vi "Read_Write_Template.vi"(0 "Template File":path, 1 "Mode":T1, 5 "Channel names In":string[](array[string]), 7 "Single Value In":string, 9 "2D Info In":string[][](array[string]), 11 "1D Info In":string[](array[string]), 12 "Save file":bool=TRUE, 13 "Data type":string="Tolerance") -> (3 "Freshly Loaded?":bool, 4 "Template File Out":path, 6 "Template Ch Names Out":string[](array[string]), 8 "Single Value Out":string, 10 "2D Info Out":string[][](array[string]), 14 "Template Info":string[][](array[string]), 15 "1D Info Out":string[](array[string]))   [LabVIEW 2011]
uses:
  Controls/Global_mode.ctl
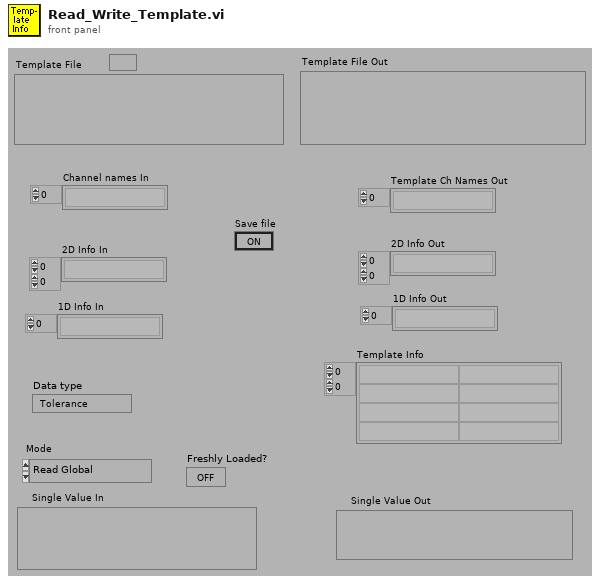
[diagram p1: front panel]
types:
  T1 = typedef "Global_mode.ctl" = enum16{"Read Global", "Load Global From File", "Write Global to File"}
  T2 = typedef "File_Status.ctl" = enum16{"Invalid Path", "This is a folder pathname", "Generic File Error", "Directory structure cannot be created", "File cannot be created", "File can be created", "File exist but read only", "File exist but no access", "File exist with read and write access"}
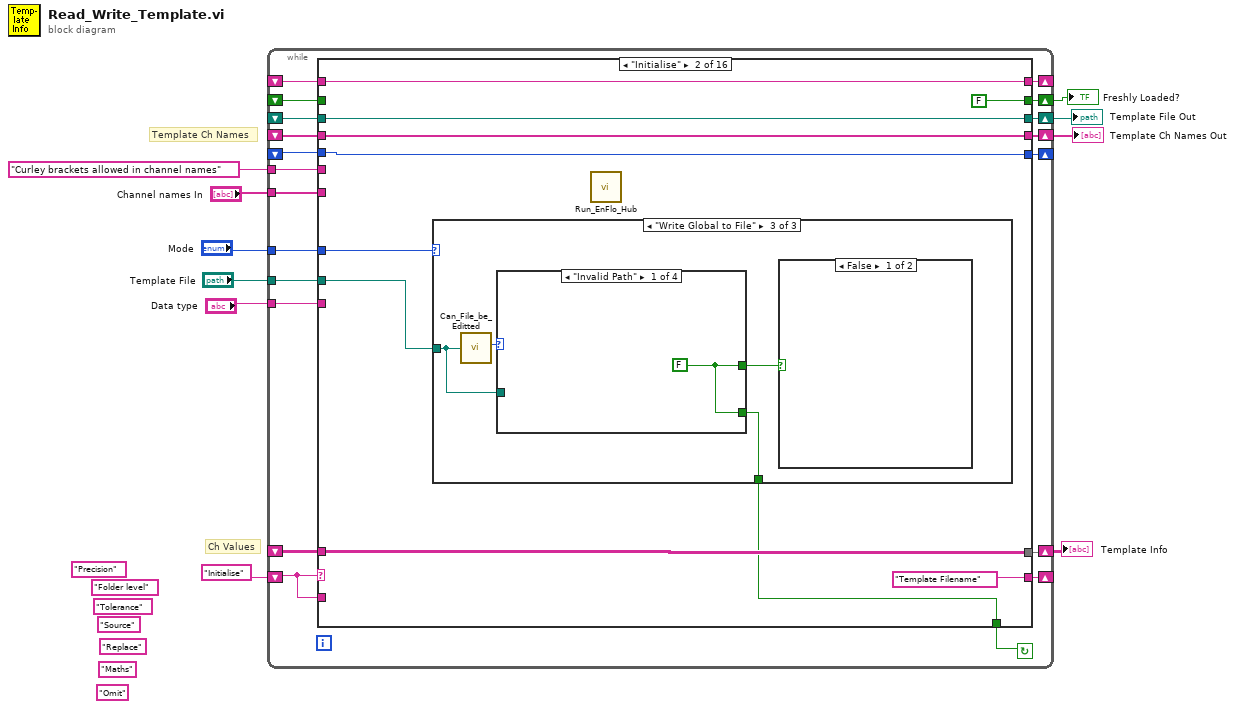
[diagram p0: block diagram]
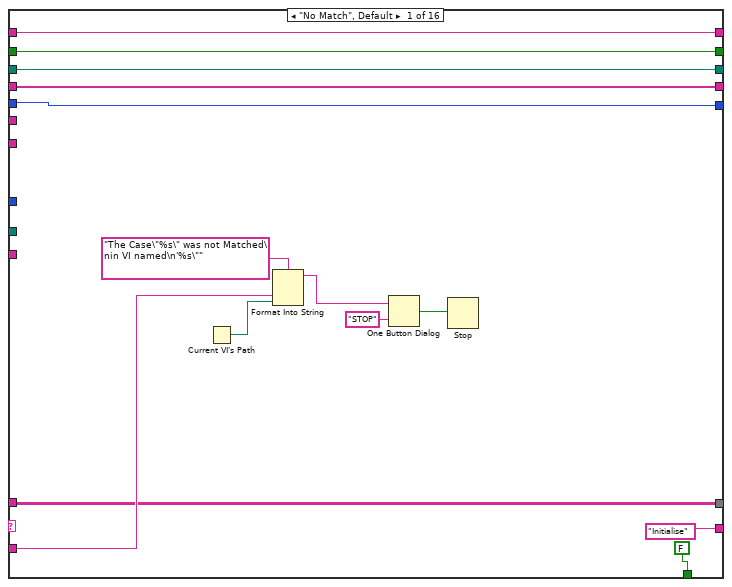
[diagram p2: hidden frame]
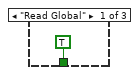
[diagram p3: hidden frame]
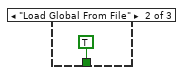
[diagram p4: hidden frame]
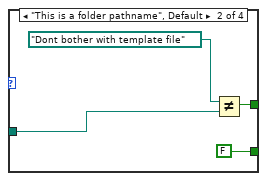
[diagram p5: hidden frame]
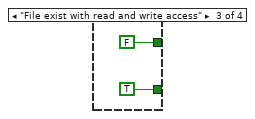
[diagram p6: hidden frame]
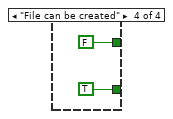
[diagram p7: hidden frame]
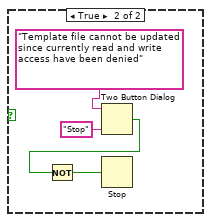
[diagram p8: hidden frame]
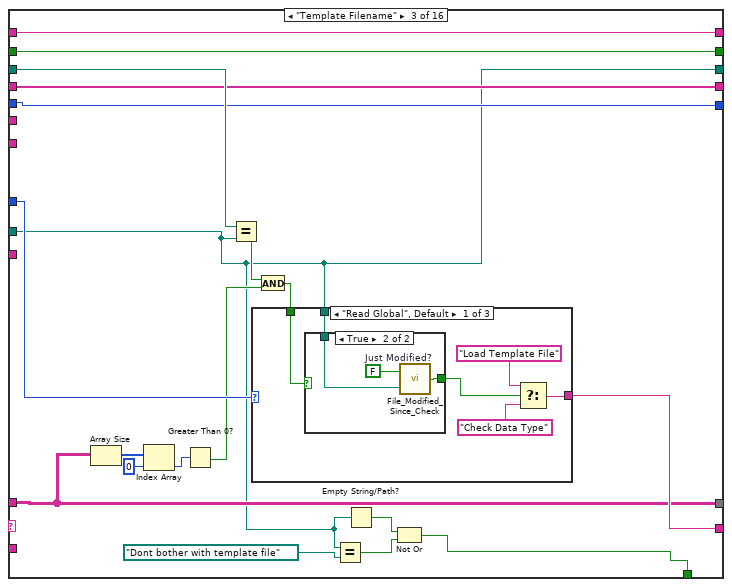
[diagram p9: hidden frame]
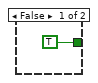
[diagram p10: hidden frame]
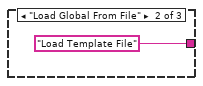
[diagram p11: hidden frame]
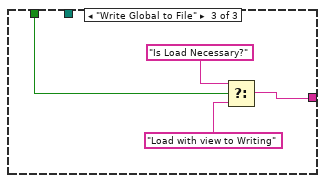
[diagram p12: hidden frame]
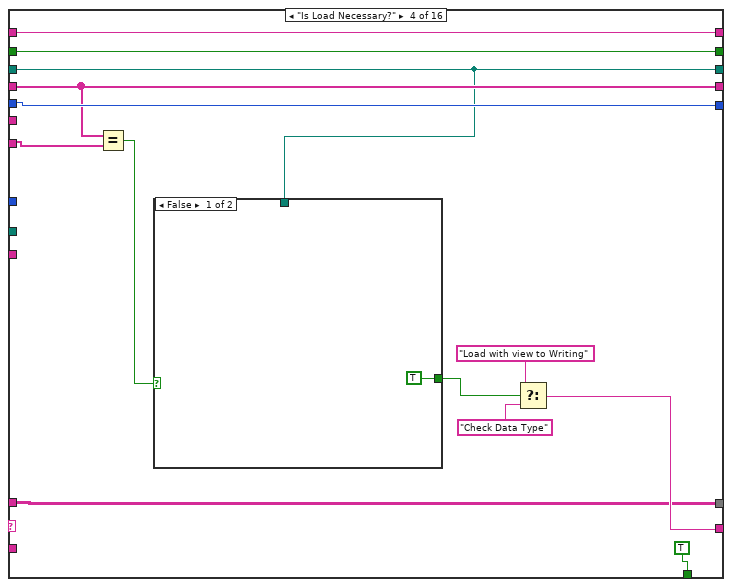
[diagram p13: hidden frame]
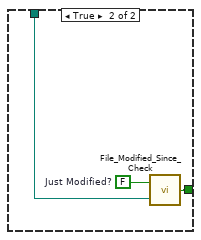
[diagram p14: hidden frame]
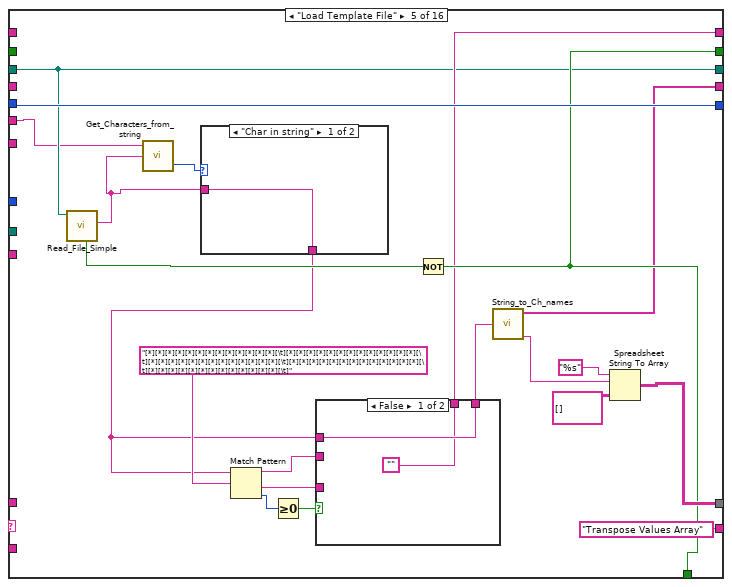
[diagram p15: hidden frame]
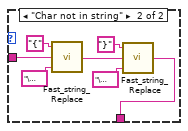
[diagram p16: hidden frame]
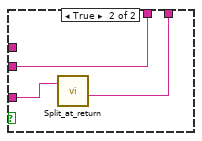
[diagram p17: hidden frame]
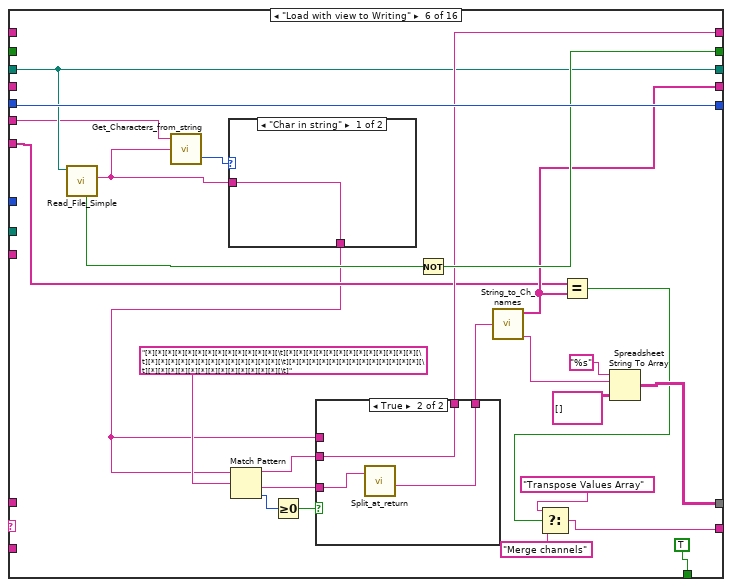
[diagram p18: hidden frame]
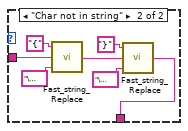
[diagram p19: hidden frame]
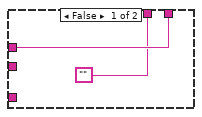
[diagram p20: hidden frame]
diagram:
  (unwired) "Precision"
  (unwired) "Folder level"
  (unwired) "Omit"
  (unwired) "Maths"
  (unwired) "Tolerance"
  (unwired) "Source"
  (unwired) "Replace"
  # "Template Ch Names"
  # "Ch Values"
  n1 = while {
    shift-left: _ -> [w15]
    shift-right: [w16] -> w3
    tunnel: "Channel names In" -> [w18]
    shift-left: _ -> [w17]
    shift-right: [w19] -> _
    tunnel: "Data type" -> [w20]
    shift-left: _ -> [w21]
    shift-right: [w22] -> w6
    shift-left: _ -> [w25]
    shift-right: [w24] -> w7
    shift-left: _ -> [w26]
    shift-right: [w27] -> w8
    tunnel: "Mode" -> [w28]
    shift-left: "Initialise" -> [w23]
    shift-right: [w29] -> _
    shift-right: [w14] -> _
    shift-left: _ -> [w13]
    tunnel: "Template File" -> [w12]
    tunnel: "Curley brackets allowed in channel names" -> [w11]
    stop <- w30 continue-if-true
    n2 = case shown="\"Initialise\"" w23 {
      tunnel: [FALSE w45 w75 TRUE w138 TRUE ("Save file") TRUE ("Save file") TRUE w243 FALSE FALSE FALSE "Save file" FALSE ("Save file") w472 FALSE] -> w30
      tunnel: ["Initialise" "Template Filename" w89 w120 "Transpose Values Array" w166 "Transpose Values Array" "Check Data Type" w240 "" "" "" "Save Template File" "End" w469 "End"] -> w29
      tunnel: w28 -> [_ w47 w90 _ _ _ _ _ w242 _ _ _ _ _ _ _]
      tunnel: [w35 w53 w85 w114 w142 w182 w203 w230 w246 w310 w324 w344 w370 w457 w467 w526] -> w27
      tunnel: w26 -> [w35 w53 w85 w114 _ _ w201 w229 w246 w310 w324 w344 w371 w457 w466 w526]
      tunnel: w25 -> [w37 w54 w92 w110 w130 w163 w206 w225 w245 w312 w330 w346 w372 w451 w471 w525]
      tunnel: [w37 w54 w74 w110 w130 w163 w206 w225 w245 w312 w330 w346 w372 w451 w471 w525] -> w24
      tunnel: w23 -> [w39 _ _ _ _ _ _ _ _ _ _ _ _ _ _ _]
      tunnel: [w38 w52 w91 w113 w129 w170 w205 w224 w244 w308 w325 w341 w365 w460 w470 w524] -> w22
      tunnel: w21 -> [w38 w52 w91 w113 _ _ w204 w224 w244 w308 w325 w341 w365 w460 w470 w524]
      tunnel: w20 -> [_ _ _ _ _ _ _ _ w247 w311 w322 w345 w368 w453 _ _]
      tunnel: [w33 w50 w84 w118 w144 w184 w209 w223 w241 w301 w327 w333 w363 w459 w468 w522] -> w19
      tunnel: w18 -> [_ _ _ w112 _ w169 w205 _ _ w302 _ w338 w364 _ _ _]
      tunnel: w17 -> [w33 w50 w84 w118 w144 w184 w209 w223 _ w301 w327 w333 w363 w459 w468 w522]
      tunnel: [w32 FALSE w80 w109 w138 w178 w207 w221 w239 w300 w326 w332 w362 w458 w465 w520] -> w16
      tunnel: w15 -> [w32 _ w80 w109 _ _ w207 w221 w239 w300 w326 w332 w362 w458 w465 w520]
      tunnel: [w31 w48 w79 w108 w132 w172 w208 w220 w238 w299 w323 w331 w360 w455 w463 w519] -> w14
      tunnel: w13 -> [w31 w48 w79 w108 _ _ w208 w220 w238 w299 w323 w331 w360 w454 w464 w519]
      tunnel: w12 -> [_ w46 w74 _ _ _ _ _ _ _ _ _ _ _ _ _]
      tunnel: w11 -> [_ _ _ _ w126 w162 _ _ _ _ _ _ _ _ w462 _]
      frame "No Match", Default {
        n3 = Current VI's Path() -> (path=w40:path)
        n4 = Format Into String(format string="The Case\"%s\" was not Matched\nin VI named\n'%s\"" ("Format String"), w39, w40) -> (resulting string=w43:string)  [unwired: 2 in, 1 out]
        n5 = One Button Dialog(message=w43, button name ("OK")="STOP") -> (true=w41:bool)
        n6 = Stop(stop? (T)=w41) -> ()
      }
      frame "Initialise" {
        n7 = case shown="\"Write Global to File\"" w47 {
          tunnel: w46 -> [_ _ w57]
          tunnel: [TRUE TRUE w58] -> w45
          frame "Read Global" {
          }
          frame "Load Global From File" {
          }
          frame "Write Global to File" {
            n8 = call "Can_File_be_Editted.vi"("Filename"=w57) -> ("File Status"=w60:T2)  [unwired: 3 out]
            n9 = case shown="\"Invalid Path\"" w60 {
              tunnel: [w61 w63 FALSE FALSE] -> w59
              tunnel: [w61 FALSE TRUE TRUE] -> w58
              tunnel: w57 -> [_ w62 _ _]
              frame "Invalid Path" {
                w61 = FALSE
              }
              frame "This is a folder pathname", Default {
                n10 = Not Equal?(x=path "Dont bother with template file" ("Template File"), y=w62) -> (x != y?=w63:bool)
              }
              frame "File exist with read and write access" {
              }
              frame "File can be created" {
              }
            }
            n11 = case shown="False" w59 {
              frame False {
              }
              frame True {
                n12 = Two Button Dialog(message="Template file cannot be updated since currently read and write access have been denied", 1:"Stop" ("F button name (\"Cancel\")")) -> (T button?=w71:bool)  [unwired: 1 out]
                n13 = Not(x=w71) -> (.not. x?=w70:bool)
                n14 = Stop(stop? (T)=w70) -> ()
              }
            }
          }
        }
        n15 = call "Run_EnFlo_Hub.vi"() -> ()  [unwired: 8 out]
      }
      frame "Template Filename" {
        n16 = Array Size(array=w85) -> (size(s)=w86:i32[])
        n17 = Index Array(array=w86, index=0 ("Index")) -> (element=w88:i32)
        n18 = Greater Than 0?(x=w88) -> (x > 0?=w81:bool)
        n19 = Equal?(x=w92, y=w74) -> (x = y?=w83:bool)
        n20 = And(x=w83, y=w81) -> (x .and. y?=w82:bool)
        n21 = case shown="\"Read Global\", Default" w90 {
          tunnel: w82 -> [w98 _ w107]
          tunnel: [w94 "Load Template File" w105] -> w89
          tunnel: w74 -> [w97 _ _]
          frame "Read Global", Default {
            n22 = case shown="True" w98 {
              tunnel: w97 -> [_ w102]
              tunnel: [TRUE ("Modified?") w101] -> w96
              frame False {
              }
              frame True {
                w100 = FALSE  # Just Modified?
                n23 = call "File_Modified_Since_Check.vi"("Pathname"=w102, "Just Modified?"=w100) -> ("Modified?"=w101:bool)
              }
            }
            n24 = Select(t="Load Template File", s=w96, f="Check Data Type") -> (s? t:f=w94:string)
          }
          frame "Load Global From File" {
          }
          frame "Write Global to File" {
            n25 = Select(t="Is Load Necessary?", s=w107, f="Load with view to Writing") -> (s? t:f=w105:string)
          }
        }
        n26 = Equal?(x=w74, y=path "Dont bother with template file" ("Template File")) -> (x = y?=w77:bool)
        n27 = Empty String/Path?(string/path=w74) -> (empty?=w76:bool)
        n28 = Not Or(1:w77, 2:w76) -> (0:w75:bool)
      }
      frame "Is Load Necessary?" {
        n29 = Equal?(x=w113, y=w112) -> (x = y?=w111:bool)
        n30 = case shown="False" w111 {
          tunnel: w110 -> [_ w124]
          tunnel: [TRUE ("Modified?") w123] -> w117
          frame False {
          }
          frame True {
            w122 = FALSE  # Just Modified?
            n31 = call "File_Modified_Since_Check.vi"("Pathname"=w124, "Just Modified?"=w122) -> ("Modified?"=w123:bool)
          }
        }
        n32 = Select(t="Load with view to Writing", s=w117, f="Check Data Type") -> (s? t:f=w120:string)
      }
      frame "Load Template File" {
        n33 = call "Read_File_Simple.vi"("Filename"=w130) -> ("Error?"=w143:bool, "string"=w127:string)  [unwired: 2 in, 6 out]
        n34 = call "Get_Characters_from_string.vi"("Input string"=w127, "Variable name"=w126) -> ("Status"=w128:enum16{"Char in string", "Char not in string"})  [unwired: 1 in, 1 out]
        n35 = case shown="\"Char in string\"" w128 {
          tunnel: w127 -> [w146 w152]
          tunnel: [w146 w147] -> w125
          frame "Char in string" {
          }
          frame "Char not in string" {
            n36 = call "Fast_string_Replace.vi"("Replace match with:"="\u0002" ("regular expression"), "Input String"=w152, "regular expression"="{") -> ("Output String"=w148:string)  [unwired: 2 out]
            n37 = call "Fast_string_Replace.vi"("Replace match with:"="\u0003" ("regular expression"), "Input String"=w148, "regular expression"="}") -> ("Output String"=w147:string)  [unwired: 2 out]
          }
        }
        n38 = Match Pattern(string=w125, regular expression="[*][*][*][*][*][*][*][*][*][*][*][*][*][\t][*][*][*][*][*][*][*][*][*][*][*][*][*][\t][*][*][*][*][*][*][*][*][*][*][*][*][*][\t][*][*][*][*][*][*][*][*][*][*][*][*][*][\t][*][*][*][*][*][*][*][*][*][*][*][*][*][\t]" ("String")) -> (before substring=w131:string, after substring=w136:string, offset past match=w135:i32)  [unwired: 2 out]
        n39 = Greater Or Equal To 0?(x=w135) -> (x >= 0?=w134:bool)
        n40 = case shown="False" w134 {
          tunnel: w136 -> [_ w158]
          tunnel: [w155 w157] -> w133
          tunnel: w125 -> [w155 _]
          tunnel: ["" w156] -> w132
          tunnel: w131 -> [_ w156]
          frame False {
          }
          frame True {
            n41 = call "Split_at_return.vi"("String"=w158) -> ("after substring"=w157:string)  [unwired: 1 in, 3 out]
          }
        }
        n42 = Not(x=w143) -> (.not. x?=w138:bool)
        n43 = call "String_to_Ch_names.vi"("Spreadsheet string"=w133) -> ("Ch names"=w129:string[], "String After names"=w139:string)  [unwired: 2 out]
        n44 = Spreadsheet String To Array(format string="%s", spreadsheet string=w139, array type (2D Dbl)=string[][] [] ("Channel Values")) -> (array=w142:string[][])  [unwired: 1 out]
      }
      frame "Load with view to Writing" {
        n45 = call "Read_File_Simple.vi"("Filename"=w163) -> ("Error?"=w183:bool, "string"=w160:string)  [unwired: 2 in, 6 out]
        n46 = call "Get_Characters_from_string.vi"("Input string"=w160, "Variable name"=w162) -> ("Status"=w161:enum16{"Char in string", "Char not in string"})  [unwired: 1 in, 1 out]
        n47 = case shown="\"Char in string\"" w161 {
          tunnel: w160 -> [w185 w191]
          tunnel: [w185 w186] -> w159
          frame "Char in string" {
          }
          frame "Char not in string" {
            n48 = call "Fast_string_Replace.vi"("Replace match with:"="\u0002" ("regular expression"), "Input String"=w191, "regular expression"="{") -> ("Output String"=w187:string)  [unwired: 2 out]
            n49 = call "Fast_string_Replace.vi"("Replace match with:"="\u0003" ("regular expression"), "Input String"=w187, "regular expression"="}") -> ("Output String"=w186:string)  [unwired: 2 out]
          }
        }
        n50 = Match Pattern(string=w159, regular expression="[*][*][*][*][*][*][*][*][*][*][*][*][*][\t][*][*][*][*][*][*][*][*][*][*][*][*][*][\t][*][*][*][*][*][*][*][*][*][*][*][*][*][\t][*][*][*][*][*][*][*][*][*][*][*][*][*][\t][*][*][*][*][*][*][*][*][*][*][*][*][*][\t]" ("String")) -> (before substring=w171:string, after substring=w176:string, offset past match=w175:i32)  [unwired: 2 out]
        n51 = Greater Or Equal To 0?(x=w175) -> (x >= 0?=w174:bool)
        n52 = case shown="True" w174 {
          tunnel: w176 -> [_ w197]
          tunnel: [w194 w196] -> w173
          tunnel: w159 -> [w194 _]
          tunnel: ["" w195] -> w172
          tunnel: w171 -> [_ w195]
          frame False {
          }
          frame True {
            n53 = call "Split_at_return.vi"("String"=w197) -> ("after substring"=w196:string)  [unwired: 1 in, 3 out]
          }
        }
        n54 = Not(x=w183) -> (.not. x?=w178:bool)
        n55 = call "String_to_Ch_names.vi"("Spreadsheet string"=w173) -> ("Ch names"=w170:string[], "String After names"=w179:string)  [unwired: 2 out]
        n56 = Equal?(x=w169, y=w170) -> (x = y?=w168:bool)
        n57 = Select(t="Transpose Values Array", s=w168, f="Merge channels") -> (s? t:f=w166:string)
        n58 = Spreadsheet String To Array(format string="%s", spreadsheet string=w179, array type (2D Dbl)=string[][] [] ("Channel Values")) -> (array=w182:string[][])  [unwired: 1 out]
      }
      frame "Merge channels" {
        n59 = Array Size(array=w201) -> (size(s)=w200:i32[])
        n60 = Index Array(array=w200, index=0) -> (element=w198:i32)
        n61 = case shown="1, Default" w198 {
          tunnel: w205 -> [w212 w219]
          tunnel: w204 -> [_ w218]
          tunnel: w201 -> [_ w217]
          tunnel: [w211 w216] -> w203
          frame 0 {
            n62 = Array Size(array=w212) -> (size(s)=w213:i32)
            n63 = Initialize Array("", 0 ("Dimension Size"), w213) -> (w211:string[][])
          }
          frame 1, Default {
            n64 = call "Merge_2D_values.vi"("Values In"=w217, "Present Channels"=w218, "Desired Channels"=w219) -> ("Values Out"=w216:string[][])
          }
        }
      }
      frame "Transpose Values Array" {
        n65 = Array Size(array=w229) -> (size(s)=w227:i32[])
        n66 = Index Array(array=w227, index=1 ("Index")) -> (element=w226:i32)
        n67 = for {
          N: w226 -> [_]
          tunnel: w229 -> [w234]
          tunnel: [w235] -> w230 mode=indexing
          i -> [w233]
          n68 = Index Array(array=w234, index (col)=w233) -> (element=w232:string[])  [unwired: 1 in]
          n69 = for {
            tunnel: [w237] -> w235 mode=indexing
            tunnel: w232 -> [w236] mode=indexing
            n70 = call "Remove_Quotes.vi"("String"=w236) -> ("String Out"=w237:string)
          }
        }
      }
      frame "Check Data Type" {
        n71 = case shown="\"Precision\"" w247 {
          tunnel: [1 1 1 1 1 2 1 1 2 2 2 1 2 1 1 0] -> w241
          tunnel: w247 -> [w258 _ _ _ _ _ _ _ _ _ _ _ _ _ _ _]
          tunnel: [w257 TRUE TRUE TRUE TRUE TRUE TRUE TRUE TRUE TRUE TRUE TRUE TRUE TRUE TRUE TRUE] -> w243
          frame "No Match", Default {
            n72 = Empty String/Path?(string/path=w258) -> (empty?=w259:bool)
            n73 = case shown="False" w259 {
              tunnel: w258 -> [w262 _]
              tunnel: [FALSE FALSE] -> w257
              frame False {
                n74 = Current VI's Path() -> (path=w263:path)
                n75 = Format Into String(format string="The Case\"%s\" was not Matched\nin VI named\n'%s\"" ("Format String"), w262, w263) -> (resulting string=w266:string)  [unwired: 2 in, 1 out]
                n76 = One Button Dialog(message=w266, button name ("OK")="STOP") -> (true=w264:bool)
                n77 = Stop(stop? (T)=w264) -> ()
              }
              frame True {
              }
            }
          }
          frame "Description" {
          }
          frame "Dispose" {
          }
          frame "Decimal" {
          }
          frame "Precision" {
          }
          frame "Multiple Sources" {
          }
          frame "Summarise" {
          }
          frame "Tolerance" {
          }
          frame "Source" {
          }
          frame "Replace" {
          }
          frame "Ignore When" {
          }
          frame "Maths" {
          }
          frame "Omit" {
          }
          frame "Folder level" {
          }
          frame "Minimum Value" {
          }
          frame "Log Folder Name" {
          }
        }
        n78 = case shown="\"Write Global to File\"" w242 {
          tunnel: w241 -> [w249 w253]
          tunnel: [w248 w254] -> w240
          frame "Read Global", Default {
            n79 = case shown="0" w249 {
              tunnel: ["Create Outputs 2D" "Create Outputs 1D" "Create single value output"] -> w248
              frame 2, Default {
              }
              frame 1 {
              }
              frame 0 {
              }
            }
          }
          frame "Write Global to File" {
            n80 = case shown="0" w253 {
              tunnel: ["Replace single value" "Replace Values"] -> w254
              frame 0 {
              }
              frame 1, Default {
              }
            }
          }
        }
      }
      frame "Create Outputs 1D" {
        n81 = for {
          tunnel: w311 -> [w320]
          tunnel: w310 -> [w319] mode=indexing
          tunnel: [w318] -> w309 mode=indexing
          n82 = call "Get_Array_Subset.vi"("String Array In"=w319, "Subset Name"=w320) -> ("First Element"=w318:string)  [unwired: 4 out]
        }
        n83 = Array Size(array=w302) -> (size(s)=w304:i32)
        n84 = Equal To 0?(x=w304) -> (x = 0?=w303:bool)
        n85 = case shown="False" w303 {
          tunnel: w309 -> [w316 w317]
          tunnel: w302 -> [w315 _]
          tunnel: w308 -> [w314 _]
          tunnel: [w313 w317] -> w307
          frame False {
            n86 = call "Merge_row_values.vi"("Present Row values"=w316, "Present Channels"=w314, "Desired Channels"=w315) -> ("Desired Row values"=w313:string[])  [unwired: 1 out]
          }
          frame True {
          }
        }
        "1D Info Out" <- w307
      }
      frame "Create single value output" {
        n87 = call "Get_Characters_from_string.vi"("Input string"=w323, "Variable name"=w322) -> ("Value"=→"Single Value Out":string)  [unwired: 1 in, 1 out]
      }
      frame "Create Outputs 2D" {
        n88 = for {
          tunnel: w345 -> [w359]
          tunnel: w344 -> [w358] mode=indexing
          tunnel: [w357] -> w340 mode=indexing
          n89 = call "Get_Array_Subset.vi"("String Array In"=w358, "Subset Name"=w359) -> ("Array Subset Out"=w357:string[])  [unwired: 4 out]
        }
        n90 = Equal?(x=w341, y=w338) -> (x = y?=w336:bool)
        n91 = Array Size(array=w338) -> (size(s)=w337:i32)
        n92 = Equal To 0?(x=w337) -> (x = 0?=w335:bool)
        n93 = Or(x=w336, y=w335) -> (x .or. y?=w334:bool)
        n94 = case shown="False" w334 {
          tunnel: w341 -> [w350 _]
          tunnel: w338 -> [w349 _]
          tunnel: w340 -> [w348 w356]
          tunnel: [w347 w356] -> w339
          frame False {
            n95 = for {
              tunnel: w350 -> [w355]
              tunnel: w349 -> [w354] mode=indexing
              tunnel: w348 -> [w352]
              tunnel: [w351] -> w347 mode=indexing
              n96 = Search 1D Array(1D array=w355, element=w354) -> (index of element=w353:i32)  [unwired: 1 out]
              n97 = Index Array(array=w352, index (row)=w353) -> (element=w351:string[])  [unwired: 1 in]
            }
          }
          frame True {
          }
        }
        "2D Info Out" <- w339
      }
      frame "Replace Values" {
        n98 = for {
          tunnel: w368 -> [w381]
          tunnel: w371 -> [w380] mode=indexing
          tunnel: [w379] -> w370 mode=indexing
          tunnel: w365 -> [w378] mode=indexing
          tunnel: w363 -> [w377]
          tunnel: "1D Info In" -> [w376]
          tunnel: "2D Info In" -> [w375]
          tunnel: w365 -> [w374] mode=indexing
          tunnel: w364 -> [w373]
          n99 = stacked-sequence {
            seq-local: [_ w391 _ _ _] -> [_ _ _ w442 _]
            seq-local: [_ w390 _ _ _] -> [_ _ _ w443 _]
            seq-local: [_ _ w402 _ _] -> [_ _ _ w441 _]
            seq-local: [_ w389 _ _ _] -> [_ _ w398 _ _]
            seq-local: [w384 _ _ _ _] -> [_ _ w399 _ _]
            seq-local: [w382 _ _ _ _] -> [_ _ w397 _ _]
            tunnel: w381 -> [_ w396 _ w444 _]
            tunnel: w380 -> [_ w393 _ _ _]
            tunnel: [_ _ _ w434 _] -> w379
            tunnel: w378 -> [_ _ _ w435 _]
            tunnel: w377 -> [w383 _ _ _ _]
            tunnel: w376 -> [_ _ w401 _ _]
            tunnel: w375 -> [_ _ w400 _ _]
            tunnel: w374 -> [w386 _ _ _ _]
            tunnel: w373 -> [w385 _ _ _ _]
            frame #0 {
              n100 = Search 1D Array(1D array=w385, element=w386) -> (index of element=w382:i32)  [unwired: 1 out]
              n101 = case shown="-1" w382 {
                tunnel: [w387 0] -> w384
                tunnel: w383 -> [w387 _]
                frame 0, Default {
                }
                frame -1 {
                }
              }
            }
            frame #1 {
              n102 = call "Get_Array_Subset.vi"("String Array In"=w393, "Subset Name"=w396) -> ("index after match"=w392:i32, "Array Subset Out"=w389:string[], "Length before match"=w394:i32)  [unwired: 2 out]
              n103 = Array Subset(array=w393, index=0 ("Array Index"), length=w394) -> (w391:string[])
              n104 = Array Subset(array=w393, index=w392) -> (w390:string[])  [unwired: 1 in]
            }
            frame #2 {
              n105 = case shown="2, Default" w399 {
                tunnel: [w406 w430 w433] -> w402
                tunnel: w401 -> [_ w432 _]
                tunnel: w400 -> [w405 _ _]
                tunnel: w398 -> [_ _ w433]
                tunnel: w397 -> [w403 w429 _]
                frame 2, Default {
                  n106 = Index Array(array=w405, index (row)=w403) -> (element=w404:string[])  [unwired: 1 in]
                  n107 = while {
                    shift-left: _ -> [w407]
                    shift-right: [w408] -> _
                    tunnel: [w409] -> w406
                    tunnel: w404 -> [w411]
                    i -> [w412]
                    stop <- w410 continue-if-true
                    n108 = case shown="0, Default" w412 {
                      tunnel: w411 -> [w414 w417]
                      tunnel: [w415 FALSE] -> w410
                      tunnel: [w414 w420] -> w409
                      tunnel: [w413 w419] -> w408
                      tunnel: w407 -> [_ w419]
                      frame 0, Default {
                        n109 = Empty String/Path?(string/path=w414) -> (empty?=w413:bool[])
                        n110 = Or Array Elements(Boolean array=w413) -> (logical OR=w415:bool)
                      }
                      frame 1 {
                        n111 = for {
                          shift-right: [w423] -> w420
                          shift-left: string[] [] -> [w422]
                          tunnel: w419 -> [w424] mode=indexing
                          tunnel: w417 -> [w421] mode=indexing
                          n112 = case shown="True" w424 {
                            tunnel: [w426 w428] -> w423
                            tunnel: w422 -> [w427 w428]
                            tunnel: w421 -> [w425 _]
                            frame False {
                              n113 = Build Array (concatenate)(w427, w425) -> (w426:string[])
                            }
                            frame True {
                            }
                          }
                        }
                      }
                    }
                  }
                }
                frame 1 {
                  n114 = Index Array(array=w432, index=w429) -> (element=w431:string)
                  n115 = Build Array(w431) -> (w430:string[])
                }
                frame 0 {
                }
              }
            }
            frame #3 {
              w436 = ""
              n116 = Format Into String(format string="**%s Start**" ("Format String"), w444) -> (resulting string=w440:string)  [unwired: 2 in, 1 out]
              n117 = Format Into String(format string="**%s End**" ("Format String"), w444) -> (resulting string=w439:string)  [unwired: 2 in, 1 out]
              n118 = Build Array (concatenate)(w442, w440, w441, w439, w443) -> (w438:string[])
              n119 = call "Clean_Up_Template.vi"("Template Info In"=w438) -> ("Template Info Out"=w437:string[])
              n120 = Build Array (concatenate)(w436, w435, w436, w437) -> (w434:string[])
            }
            frame #4 {
            }
          }
        }
      }
      frame "Replace single value" {
        w448 = FALSE  # append to file? (new file:F)
        w449 = FALSE  # advisory dialog? (display:T)
        n121 = call "Read_File_Simple.vi"("Filename"=w451) -> ("string"=w452:string)  [unwired: 2 in, 7 out]
        n122 = call "Replace_data_in_setup_string.vi"("New data string"="Single Value In", "Input string"=w454, "Variable name"=w453) -> ("Appended string"=w455:string)
        n123 = call "Replace_data_in_setup_string.vi"("New data string"="Single Value In", "Input string"=w452, "Variable name"=w453) -> ("Appended string"=w450:string)
        n124 = call "Write_Characters_To_File.vi"("file path (dialog if empty)"=w451, "advisory dialog? (display:T)"=w449, "character string"=w450, "append to file? (new file:F)"=w448) -> ()  [unwired: 1 in, 4 out]
      }
      frame "Save Template File" {
        n125 = stacked-sequence {
          seq-local: [w478 _] -> [_ w498]
          tunnel: [_ TRUE] -> w472
          tunnel: w471 -> [_ w508]
          tunnel: w470 -> [_ w507]
          tunnel: [_ "Update last Modified VI"] -> w469
          tunnel: [_ w501] -> w467
          tunnel: w466 -> [_ w500]
          tunnel: w464 -> [w475 _]
          tunnel: [w473 _] -> w463
          tunnel: w462 -> [w476 _]
          frame #0 {
            w483 = "Log Folder Name" ("Variable name")
            n126 = call "Get_Characters_from_string.vi"("Input string"=w475, "Variable name"=w483) -> ("Status"=w484:enum16{"Char in string", "Char not in string"})  [unwired: 1 in, 1 out]
            n127 = case shown="\"Char not in string\"" w484 {
              tunnel: w483 -> [_ w497]
              tunnel: w475 -> [w491 w493]
              tunnel: [w491 w492] -> w474
              frame "Char in string" {
              }
              frame "Char not in string" {
                n128 = Default Directory() -> (w496:path)
                n129 = Path To String(path=w496) -> (string=w495:string)
                n130 = call "Characters_to_string.vi"("Characters to write"=w495, "Label for characters"=w497) -> ("Output string"=w494:string)
                n131 = Concatenate Strings(w493, w494) -> (w492:string)
              }
            }
            n132 = call "Get_Characters_from_string.vi"("Input string"=w474, "Variable name"=w476) -> ("Status"=w477:enum16{"Char in string", "Char not in string"})  [unwired: 1 in, 1 out]
            n133 = case shown="\"Char in string\"" w477 {
              tunnel: w476 -> [_ w490]
              tunnel: w474 -> [w485 w488]
              tunnel: [w485 w487] -> w473
              frame "Char in string" {
              }
              frame "Char not in string" {
                n134 = call "Characters_to_string.vi"("Characters to write"="{}", "Label for characters"=w490) -> ("Output string"=w489:string)
                n135 = Concatenate Strings(w488, w489) -> (w487:string)
              }
            }
            n136 = Initialize Array("", 10 ("Dimension Size")) -> (w482:string[])
            n137 = call "Asterisk_header.vi"("Channel names"=w482) -> ("Header string"=w479:string)
            n138 = Concatenate Strings(w473, w479) -> (w478:string)
          }
          frame #1 {
            w506 = FALSE  # exists?
            n139 = Transpose 2D Array(2D array=w500) -> (transposed array=w504:string[][])
            n140 = for {
              shift-right: [w511] -> w502
              shift-left: string[][] [] -> [w510]
              tunnel: w504 -> [w509] mode=indexing
              n141 = Equal?(x=w509, y=" ") -> (x = y?=w513:bool[])
              n142 = And Array Elements(Boolean array=w513) -> (logical AND=w512:bool)
              n143 = case shown="False" w512 {
                tunnel: [w516 w518] -> w511
                tunnel: w510 -> [w517 w518]
                tunnel: w509 -> [w515 _]
                frame False {
                  n144 = Build Array (concatenate)(w517, w515) -> (w516:string[][])
                }
                frame True {
                }
              }
            }
            n145 = Transpose 2D Array(2D array=w502) -> (transposed array=w501:string[][])
            n146 = call "Write_Ch_data_file.vi"("Header string"=w498, "exists?"=w506, "Channel Values"=w502, "Channel names"=w507, "Filename"=w508) -> ()  [unwired: 3 in, 4 out]
          }
        }
      }
      frame "Update last Modified VI" {
        w521 = TRUE  # Just Modified?
        n147 = call "File_Modified_Since_Check.vi"("Pathname"=w525, "Just Modified?"=w521) -> ()  [unwired: 1 out]
      }
    }
  }
  "Template Ch Names Out" <- w6
  "Template File Out" <- w7
  "Template Info" <- w8
  "Freshly Loaded?" <- w3
